vi "visualizacion.vi"() -> ()   [LabVIEW 2017]
uses:
  <vilib>/Instr/_visa.llb/VISA Configure Serial Port (Instr).vi
panel:
  out "Limite":bool
  out "Limite":bool
  out "Limite":bool
  out "Limite":bool
  out "Eje X":u8(slide) scale=0.0..180.0
  out "Eje Y":u8(slide) scale=0.0..180.0
  in  "Puerto del arduino":refnum<visa-resource-name>
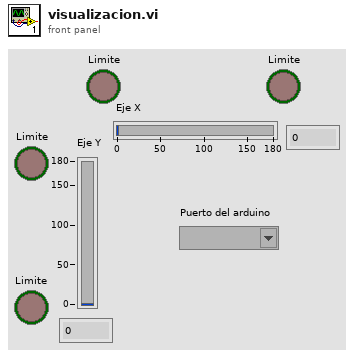
[diagram p1: front panel]
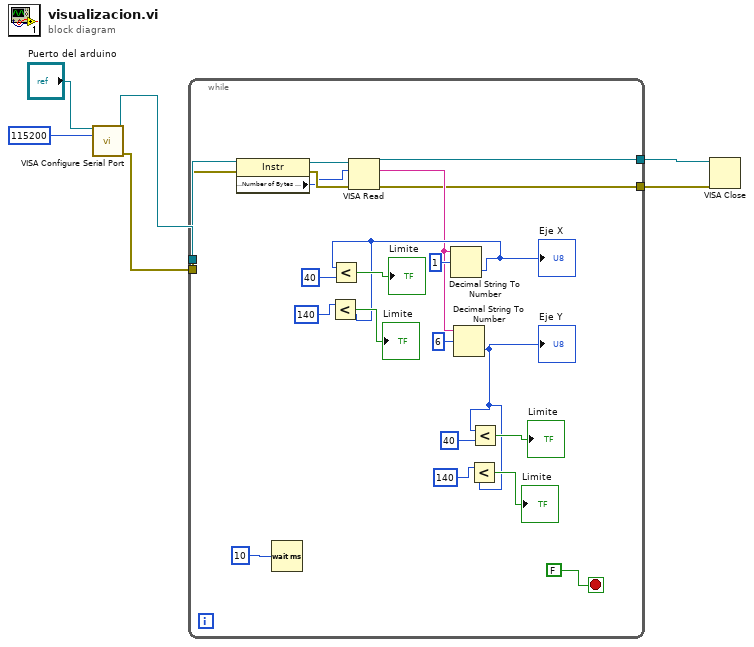
[diagram p0: block diagram]
diagram:
  n1 = call-poly "VISA Configure Serial Port"("VISA resource name"="Puerto del arduino", "baud rate (9600)"=u32 115200) -> ("VISA resource name out"=w5:refnum<visa-resource-name>, "error out"=w4:errorcluster)  [unwired: 12 in]
  n2 = while {
    tunnel: w5 -> [w28]
    tunnel: w4 -> [w26]
    tunnel: [w9] -> w2
    tunnel: [w8] -> w1
    stop <- FALSE stop-if-true
    n3 = property class="Instr"(reference=w28, error in=w26) -> (reference out=w27:refnum<visa-resource-name>, error out=w25:errorcluster, "Serial Settings:Number of Bytes at Serial Port"=w24:u32)
    n4 = Wait (ms)(milliseconds to wait=u32 10) -> ()  [unwired: 1 out]
    n5 = VISA Read(VISA resource name=w27, byte count=w24, error in (no error)=w25) -> (VISA resource name out=w9:refnum<visa-resource-name>, read buffer=w10:string, error out=w8:errorcluster)  [unwired: 1 out]
    n6 = Decimal String To Number(string=w10, offset=1) -> (number=w11:i32)  [unwired: 1 in, 1 out]
    "Eje X" <- w11
    n7 = Less?(x=140 ("y"), y=w11) -> (x < y?=→"Limite":bool)
    n8 = Less?(x=w11, y=40) -> (x < y?=→"Limite":bool)
    n9 = Decimal String To Number(string=w10, offset=6) -> (number=w13:i32)  [unwired: 1 in, 1 out]
    "Eje Y" <- w13
    n10 = Less?(x=140 ("y"), y=w13) -> (x < y?=→"Limite":bool)
    n11 = Less?(x=w13, y=40) -> (x < y?=→"Limite":bool)
  }
  n12 = VISA Close(VISA resource name=w2, error in (no error)=w1) -> ()  [unwired: 1 out]
